vi "Read ADC Response.vi"(8 "error in (no error)":errorcluster, 11 "NXP in":refnum<class "NXP.lvclass">) -> (0 "error out":errorcluster, 2 "Buffer":string, 3 "NXP out":refnum<class "NXP.lvclass">)   [LabVIEW 2020, in "NXP.lvclass"]
doc: "Método heredado del padre con un override"
uses:
  NXP.lvclass
  Abstract/Serial device/Serial device.lvclass
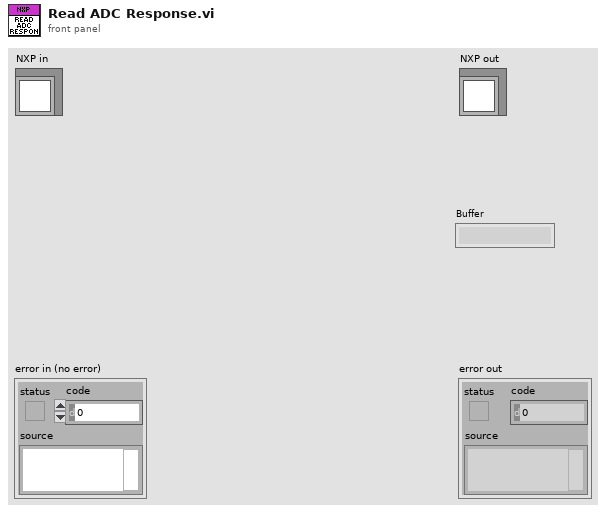
[diagram p1: front panel]
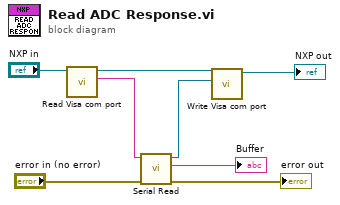
[diagram p0: block diagram]
diagram:
  n1 = call-dynamic "Read Visa com port.vi"("Serial device in"="NXP in") -> ("Visa com port"=w7:string, "Serial device out"=w6:refnum<class "NXP.lvclass">)  [unwired: 8 in, 1 out]
  n2 = call "Serial Read.vi"("error in (no error)"="error in (no error)", "VISA resource name in"=w7) -> ("error out"=→"error out":errorcluster, "Serial Response"=→"Buffer":string, "VISA resource name out"=w5:refnum<visa-resource-name>)  [unwired: 7 in]
  n3 = call-dynamic "Write Visa com port.vi"("Visa com port"=w5, "Serial device in"=w6) -> ("Serial device out"=→"NXP out":refnum<class "NXP.lvclass">)  [unwired: 8 in, 1 out]
